vi "P9P14T_Check_Queue.vi"(7 "error in (no error)":errorcluster, 10 "queue":refnum<queue>) -> (0 "error out":errorcluster, 1 "P9/P14-Magnet-Control":T1 {"Approach" items=["Linear", "NoOvershoot", "Oscillate"]}, 3 "New Entries?":bool)   [LabVIEW 2019]
uses:
  PPMS/P9P14_Magnet_Control.ctl
panel:
  out "Numeric":i32
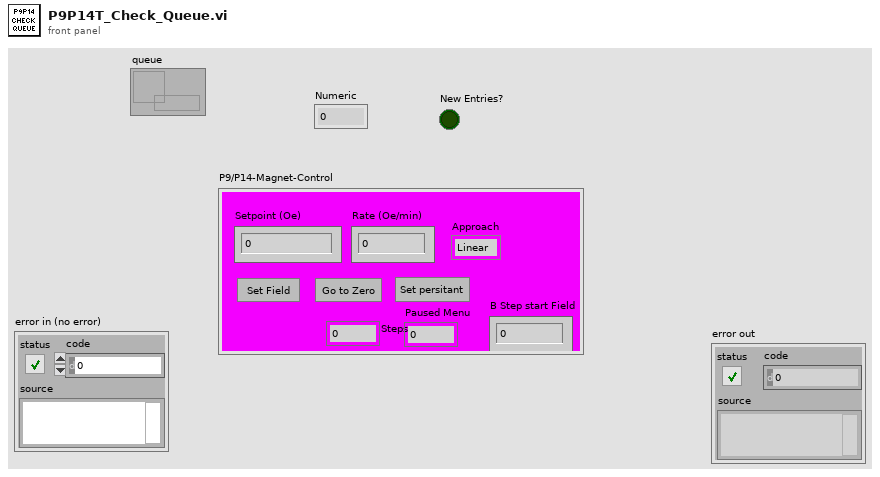
[diagram p1: front panel]
types:
  T1 = typedef "P9P14_Magnet_Control.ctl" = cluster{"Setpoint (Oe)":dbl, "Rate (Oe/min)":dbl, "Set Field":bool, "Go to zero":bool, "Set Persitant/non-pers":bool, "Approach":i32, "Steps":dbl, "Paused Menu":dbl, "B Step start Field":dbl}
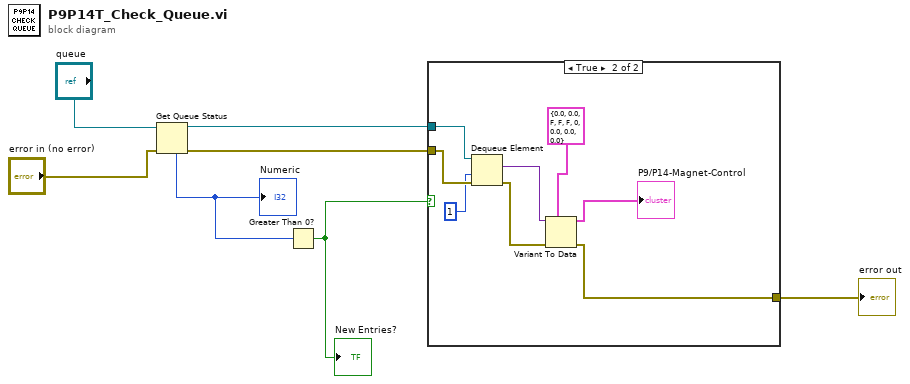
[diagram p0: block diagram]
diagram:
  n1 = Get Queue Status(queue="queue", error in (no error)="error in (no error)") -> (queue out=w3:refnum<queue>, error out=w2:errorcluster, # elements in queue=w5:i32)  [unwired: 1 in, 5 out]
  "Numeric" <- w5
  n2 = Greater Than 0?(x=w5) -> (x > 0?=w4:bool)
  "New Entries?" <- w4
  n3 = case shown="True" w4 {
    tunnel: w3 -> [_ w16]
    tunnel: w2 -> [w8 w15]
    tunnel: [w8 w11] -> w1
    frame False {
    }
    frame True {
      n4 = Dequeue Element(queue=w16, timeout in ms (-1)=1, error in (no error)=w15) -> (element=w13:variant, error out=w12:errorcluster)  [unwired: 2 out]
      n5 = Variant To Data(error in=w12, type=T1 {"Setpoint (Oe)"=0.0, "Rate (Oe/min)"=0.0, "Set Field"=FALSE, "Go to zero"=FALSE, "Set Persitant/non-pers"=FALSE, "Approach"=0, "Steps"=0.0, "Paused Menu"=0.0, "B Step start Field"=0.0} ("P9/P14-Magnet-Control"), Variant=w13) -> (data=→"P9/P14-Magnet-Control":T1, error out=w11:errorcluster)
    }
  }
  "error out" <- w1
